vi "Example - SLL CSV Logger.vi"() -> (0 "error out":errorcluster)   [LabVIEW 2014, in "SLL Spreadsheet.lvlib" / "SLL CSV Logger.lvclass"]
uses:
  SLL CSV Logger.lvclass
  SLL Spreadsheet.lvlib
panel:
  in  "2D Data with Headers":string[][](array[string])
  in  "Numeric Array Key Value Pairs":cluster{"Key":string, "Value":dbl[]}[](array[cluster])
  out "2D Array":string[][](array[string])
  in  "Key Value Pairs 2":cluster{"Key":string, "Value":string}[](array[cluster])=[{"Key"="Header 3", "Value"="333"}, {"Key"="Header 2", "Value"="222"}, {"Key"="Header 4", "Value"="444"}]
  in  "Key Value Pairs 1":cluster{"Key":string, "Value":string}[](array[cluster])=[{"Key"="Header 1", "Value"="11"}, {"Key"="Header 2", "Value"="22"}]
  in  "Headers[]":string[](array[string])=["Header 1", "Header 2", "Header 3"]
  in  "File Path":path=path "C:/Users/Public/Documents/SLL CSV Logger.csv"
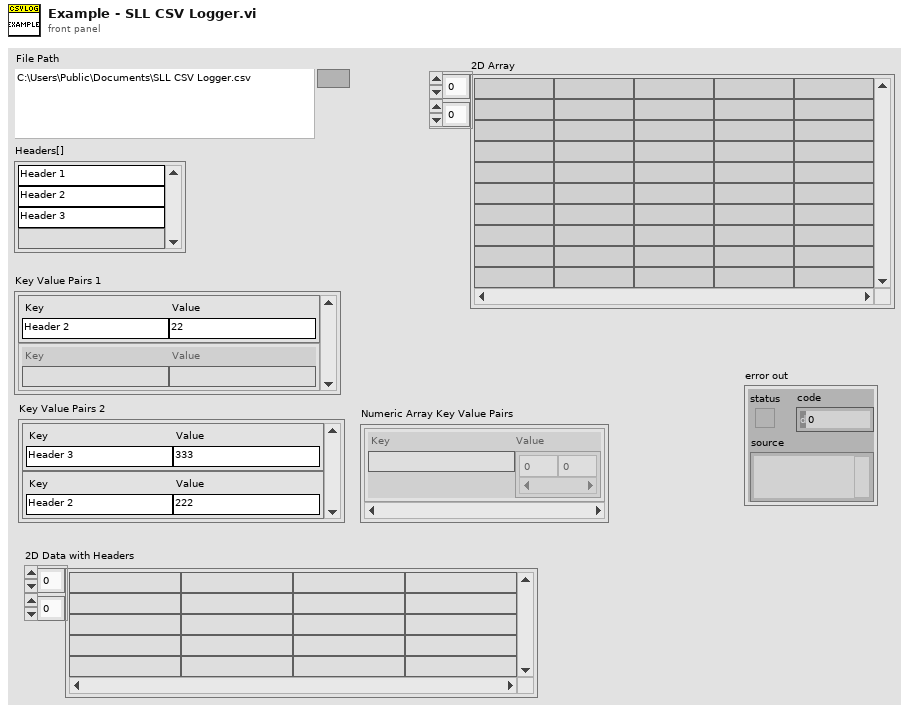
[diagram p1: front panel]
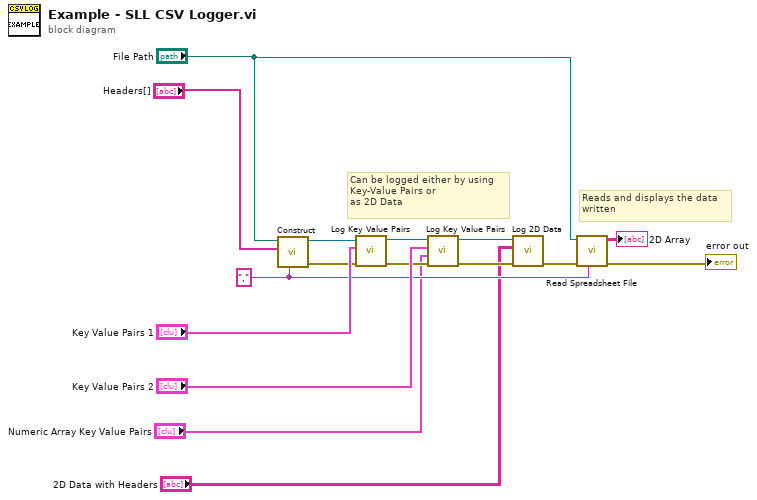
[diagram p0: block diagram]
diagram:
  w6 = "," ("Delimiter (,)")
  # "Reads and displays the data \nwritten"
  # "Can be logged either by using\nKey-Value Pairs or\nas 2D Data"
  n1 = call "Construct.vi"("Delimiter (,)"=w6, "Headers[]"="Headers[]", "File Path"="File Path") -> ("error out"=w12:errorcluster, "SLL Spreadsheet Logger out"=w11:refnum<class "SLL CSV Logger.lvclass">)  [unwired: 7 in]
  n2 = call "Log Key Value Pairs.vi"("error in (no error)"=w12, "String Key Value Pairs"="Key Value Pairs 1", "SLL Spreadsheet Logger in"=w11) -> ("error out"=w9:errorcluster, "SLL Spreadsheet Logger out"=w10:refnum<class "SLL CSV Logger.lvclass">)  [unwired: 7 in]
  n3 = call "Log Key Value Pairs.vi"("error in (no error)"=w9, "Numeric Array Key Value Pairs"="Numeric Array Key Value Pairs", "String Key Value Pairs"="Key Value Pairs 2", "SLL Spreadsheet Logger in"=w10) -> ("error out"=w16:errorcluster, "SLL Spreadsheet Logger out"=w2:refnum<class "SLL CSV Logger.lvclass">)  [unwired: 6 in]
  n4 = call "Log 2D Data.vi"("error in (no error)"=w16, "2D Data with Headers"="2D Data with Headers", "SLL Spreadsheet Logger in"=w2) -> ("error out"=w3:errorcluster)  [unwired: 7 in, 1 out]
  n5 = call "Read Spreadsheet File.vi"("Delimiter (tab)"=w6, "error in (no error)"=w3, "File Path"="File Path") -> ("error out"=→"error out":errorcluster, "2D Array"=→"2D Array":string[][])  [unwired: 7 in]
